vi "Set VI.vi"(8 "error in (no error)":errorcluster, 10 "VI ref":refnum<vi>, 11 "Deferer in":refnum<class "Deferer.lvclass">) -> (0 "error out":errorcluster)   [LabVIEW 2019, in "Panel.lvlib" / "Deferer.lvclass"]
doc: "Sets the VI associated with the deferer.\n\n----\nPlease see the following web address for additional documentation and tutorial information:\nhttp://www.mooregoodideas.com/mgi-panel-manager/\n\nAuthor: Derek Trepanier\n\nCopyright (c) 2018, Moore Good Ideas, Inc.\n\nAll rights reserved.\n\nRedistribution and use in source and binary forms, with or without modification, are permitted provided that the following conditions are met:\n\n * Redistributions of source code must retain the above copyright notice, this list of conditions and the following disclaimer.\n * Redistributions in binary form must reproduce the above copyright notice, this list of conditions and the following disclaimer in the documentation and/or other materials provided with the distribution.\n * Neither the name of Moore Good Ideas, Inc. nor the names of its contributors may be used to endorse or promote products derived from this software without specific prior written permission.\n\nTHIS SOFTWARE IS PROVIDED BY THE COPYRIGHT HOLDERS AND CONTRIBUTORS \"AS IS\" AND ANY EXPRESS OR IMPLIED WARRANTIES, INCLUDING, BUT NOT LIMITED TO, THE IMPLIED WARRANTIES OF MERCHANTABILITY AND FITNESS FOR A PARTICULAR PURPOSE ARE DISCLAIMED. IN NO EVENT SHALL THE COPYRIGHT OWNER OR CONTRIBUTORS BE LIABLE FOR ANY DIRECT, INDIRECT, INCIDENTAL, SPECIAL, EXEMPLARY, OR CONSEQUENTIAL DAMAGES (INCLUDING, BUT NOT LIMITED TO, PROCUREMENT OF SUBSTITUTE GOODS OR SERVICES; LOSS OF USE, DATA, OR PROFITS; OR BUSINESS INTERRUPTION) HOWEVER CAUSED AND ON ANY THEORY OF LIABILITY, WHETHER IN CONTRACT, STRICT LIABILITY, OR TORT (INCLUDING NEGLIGENCE OR OTHERWISE) ARISING IN ANY WAY OUT OF THE USE OF THIS SOFTWARE, EVEN IF ADVISED OF THE POSSIBILITY OF SUCH DAMAGE."
uses:
  Deferer.lvclass
  Deferer.lvclass/Deferer.ctl
  Panel Control Counter/Panel Control Counter.lvclass
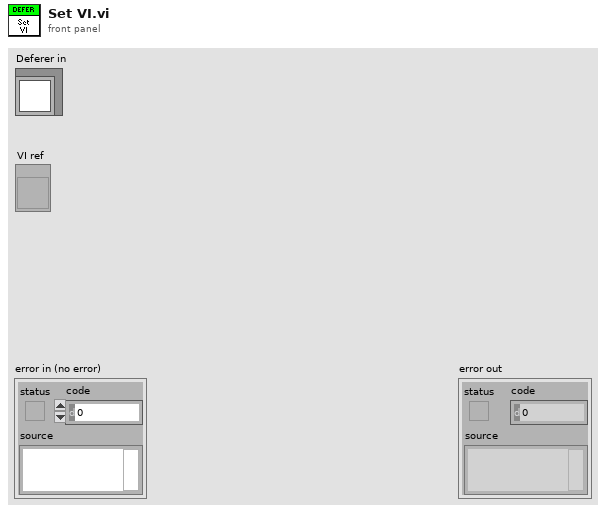
[diagram p1: front panel]
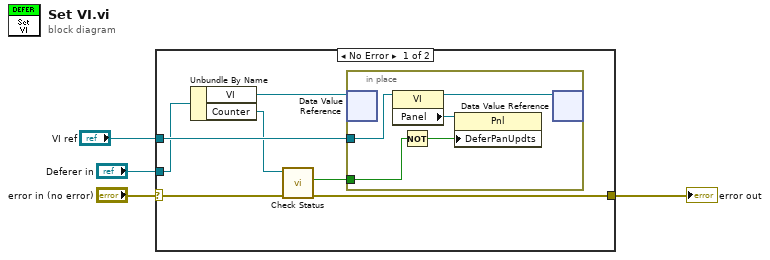
[diagram p0: block diagram]
diagram:
  n1 = case shown="No Error" "error in (no error)" {
    selector: "error in (no error)" -> [w7 w17]
    tunnel: "VI ref" -> [w10 _]
    tunnel: "Deferer in" -> [w9 _]
    tunnel: [w6 w17] -> w1
    frame No Error {
      n2 = Unbundle By Name(w9) -> ("VI"=w11:refnum<data-value>, "Counter"=w5:refnum<class "Panel Control Counter.lvclass">)
      n3 = call "Check Status.vi"("error in (no error)"=w7, "Panel Control Counter in"=w5) -> ("error out"=w6:errorcluster, "Fully Released?"=w8:bool)  [unwired: 8 in]
      n4 = in-place {
        in-place-border: w10 -> [w16]
        in-place-border: w8 -> [w13]
        n5 = in-place-dvr #1(w11) -> ()  [unwired: 2 out]
        n6 = property class="VI"(reference=w16) -> (reference out=w15:refnum<vi>, "Panel"=w14:refnum<vi>)  [unwired: 1 in, 1 out]
        n7 = Not(x=w13) -> (.not. x?=w12:bool)
        n8 = property class="Pnl"(reference=w14, "DeferPanUpdts"=w12) -> ()  [unwired: 1 in, 2 out]
        n9 = in-place-dvr #1(w15) -> ()  [unwired: 2 out]
      }
    }
    frame Error {
    }
  }
  "error out" <- w1
